vi "SeCrTs-Data reader from shared variable.vi"(0 "Data in":string, 3 "empty?":bool, 5 "error IO":errorcluster) -> (19 "error out":errorcluster)   [LabVIEW 2022 SP3]
uses:
  Globals/SeCrTS-DD globals.vi
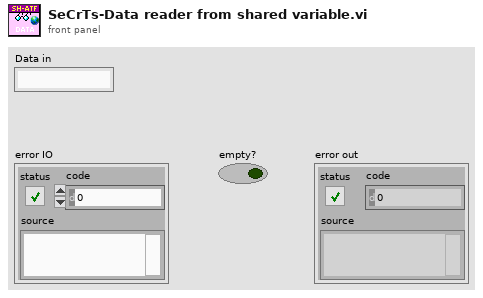
[diagram p1: front panel]
types:
  T1 = cluster{"C/NC":bool, "Start/Stop Log":bool[], "Log Name":string, "Config":cluster{"AO config":cluster{"Channel_Name":string, "Channel_Number":string, "Default_Value":dbl, "Units":string}[], "AI config":cluster{"Channel_Name":string, "Channel_Number":string, "Pre_Scale_min":dbl, "Pre_Scale_max":dbl, "Sensor_min":dbl, "Sensor_max":dbl, "Units":string}[], "DI config":cluster{"Channel_Name":string, "Channel_Number":string, "Default_Value":bool, "DI invert?":bool}[], "DO config":cluster{"Channel_Name":string, "Channel_Number":string, "Default_Value":bool, "DO invert?":bool}[], "TC config":cluster{"Channel_Name":string, "Channel_Number":string, "Pre_Scale_min":dbl, "Pre_Scale_max":dbl, "units":i32, " type":i32}[], "ACC config":cluster{"Channel_Name":string, "Channel_Number":string, "Pre_Scale_min":dbl, "Pre_Scale_max":dbl, "Terminal configuration":i32, "Sensitivity":dbl, "Sensitivity units":i32}[], "SG config":cluster{"Channel_Name":string, "Channel_Number":string, "Pre_Scale_min":dbl, "Pre_Scale_max":dbl}[], "Strain Gauge Settings":cluster{"poisson ratio":dbl, "nominal gage resistance":dbl, "gage factor":dbl}, "Bridge Settings":cluster{"voltage excitation value":dbl, "voltage excitation source":i32, "initial bridge voltage":dbl, "lead wire resistance":dbl, "strain configuration":i32}, "Sample Rate":cluster{"AI Sample Rate":dbl[], "AO Sample Rate":dbl[], "DI Sample Rate":dbl[], "TC Sample Rate":dbl[], "DO Sample Rate":dbl[], "SG Sample Rate":dbl[], "ACC Sample Rate":dbl[]}}, "Log min":dbl, "Drive":cluster{"Drive_Health":bool, "Drive_Frequency":u32, "Drive_Status":bool, "Drive_RPM":u32, "Drive_Direction":bool, "Acceleration state":bool, "Steady state":bool, "Deceleration state":bool, "Drive_Enable":bool, "Drive set_RPM":dbl}, "HOLD UPDATE":bool}
  T2 = cluster{"AO config":cluster{"Channel_Name":string, "Channel_Number":string, "Default_Value":dbl, "Units":string}[], "AI config":cluster{"Channel_Name":string, "Channel_Number":string, "Pre_Scale_min":dbl, "Pre_Scale_max":dbl, "Sensor_min":dbl, "Sensor_max":dbl, "Units":string}[], "DI config":cluster{"Channel_Name":string, "Channel_Number":string, "Default_Value":bool, "DI invert?":bool}[], "DO config":cluster{"Channel_Name":string, "Channel_Number":string, "Default_Value":bool, "DO invert?":bool}[], "TC config":cluster{"Channel_Name":string, "Channel_Number":string, "Pre_Scale_min":dbl, "Pre_Scale_max":dbl, "units":i32, " type":i32}[], "ACC config":cluster{"Channel_Name":string, "Channel_Number":string, "Pre_Scale_min":dbl, "Pre_Scale_max":dbl, "Terminal configuration":i32, "Sensitivity":dbl, "Sensitivity units":i32}[], "SG config":cluster{"Channel_Name":string, "Channel_Number":string, "Pre_Scale_min":dbl, "Pre_Scale_max":dbl}[], "Strain Gauge Settings":cluster{"poisson ratio":dbl, "nominal gage resistance":dbl, "gage factor":dbl}, "Bridge Settings":cluster{"voltage excitation value":dbl, "voltage excitation source":i32, "initial bridge voltage":dbl, "lead wire resistance":dbl, "strain configuration":i32}, "Sample Rate":cluster{"AI Sample Rate":dbl[], "AO Sample Rate":dbl[], "DI Sample Rate":dbl[], "TC Sample Rate":dbl[], "DO Sample Rate":dbl[], "SG Sample Rate":dbl[], "ACC Sample Rate":dbl[]}}
  T3 = cluster{"Drive_Health":bool, "Drive_Frequency":u32, "Drive_Status":bool, "Drive_RPM":u32, "Drive_Direction":bool, "Acceleration state":bool, "Steady state":bool, "Deceleration state":bool, "Drive_Enable":bool, "Drive set_RPM":dbl}
  T4 = cluster{"Channel names":cluster{"AI_C_Data P":string[], "AI_V_Data P":string[], "AO_Data P":string[], "DO_Data P":string[], "ACC_Data P":string[], "TC Data P":string[], "Drive_A_C":string[], "Drive_A_D":string[], "AI_C_Data S":string[], "DO_Data S":string[]}, "DI Names":cluster{"Di P":string[], "Di S":string[]}}
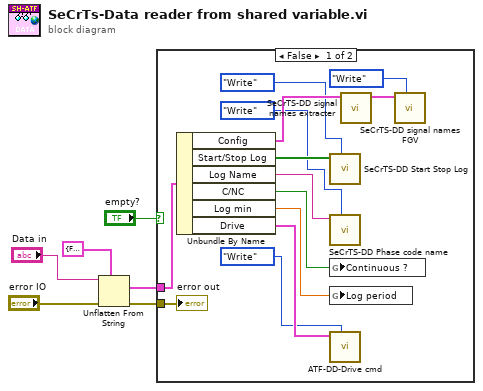
[diagram p0: block diagram]
diagram:
  n1 = Unflatten From String(type=T1 {"C/NC"=FALSE, "Start/Stop Log"=[], "Log Name"="", "Config"={"AO config"=[], "AI config"=[], "DI config"=[], "DO config"=[], "TC config"=[], "ACC config"=[], "SG config"=[], "Strain Gauge Settings"={"poisson ratio"=0.0, "nominal gage resistance"=0.0, "gage factor"=0.0}, "Bridge Settings"={"voltage excitation value"=0.0, "voltage excitation source"=0, "initial bridge voltage"=0.0, "lead wire resistance"=0.0, "strain configuration"=0}, "Sample Rate"={"AI Sample Rate"=[], "AO Sample Rate"=[], "DI Sample Rate"=[], "TC Sample Rate"=[], "DO Sample Rate"=[], "SG Sample Rate"=[], "ACC Sample Rate"=[]}}, "Log min"=0.0, "Drive"={"Drive_Health"=FALSE, "Drive_Frequency"=0, "Drive_Status"=FALSE, "Drive_RPM"=0, "Drive_Direction"=FALSE, "Acceleration state"=FALSE, "Steady state"=FALSE, "Deceleration state"=FALSE, "Drive_Enable"=FALSE, "Drive set_RPM"=0.0}, "HOLD UPDATE"=FALSE} ("notification"), binary string="Data in", error in (no error)="error IO") -> (value=w5:T1, error out=w6:errorcluster)  [unwired: 2 in, 1 out]
  n2 = case shown="False" "empty?" {
    tunnel: w6 -> [w19 _]
    tunnel: w5 -> [w18 _]
    frame False {
      n3 = Unbundle By Name(w18) -> ("Config"=w17:T2, "Start/Stop Log"=w16:bool[], "Log Name"=w15:string, "C/NC"=w14:bool, "Log min"=w13:dbl, "Drive"=w12:T3)
      n4 = call "SeCrTS-DD Start Stop Log.vi"("Enum"=enum16{"Read", "Write"}."Write", "Start Stop log"=w16) -> ()  [unwired: 8 in, 2 out]
      n5 = call "SeCrTS-DD Phase code name.vi"("Enum"=enum16{"Read", "Write"}."Write", "Phase code W"=w15) -> ()  [unwired: 8 in, 2 out]
      n6 = global write "SeCrTS-DD globals.vi" "Continuous ?"(w14) -> ()
      n7 = global write "SeCrTS-DD globals.vi" "Log period"(w13) -> ()
      n8 = call "ATF-DD-Drive cmd.vi"("Enum"=enum16{"Read", "Write"}."Write", "Data.Drive"=w12) -> ()  [unwired: 8 in, 2 out]
      n9 = call "SeCrTS-DD signal names extracter.vi"("input cluster"=w17) -> ("Signal names"=w8:T4)  [unwired: 10 in]
      n10 = call "SeCrTS-DD signal names FGV.vi"("Enum"=enum16{"Read", "Write"}."Write", "Signal names"=w8) -> ()  [unwired: 8 in, 2 out]
      "error out" <- w19
    }
    frame True {
    }
  }
